vi "实时数据查询用2小时间的数据.vi"(11 "字符串":string) -> (3 "连接的字符串":string)   [LabVIEW 2016, in "数据传输系统-04.lvlib"]
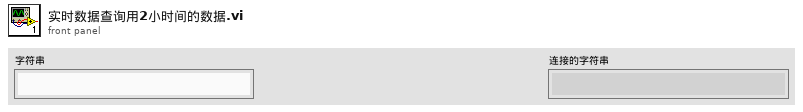
[diagram p1: front panel]
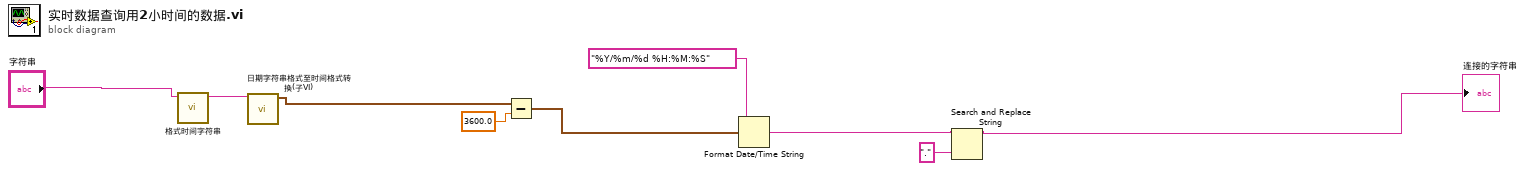
[diagram p0: block diagram]
diagram:
  n1 = call "格式时间字符串.vi"("字符串"="字符串") -> ("连接的字符串"=w2:string)  [unwired: 10 in]
  n2 = call "日期字符串格式至时间格式转换(子VI).vi"("data[0]"=w2) -> ("time stamp"=w1:timestamp)  [unwired: 10 in]
  n3 = Subtract(x=w1, y=3600.0) -> (x-y=w6:timestamp)
  n4 = Format Date/Time String(time format string (%c)="%Y/%m/%d %H:%M:%S" ("格式字符串"), seconds (now)=w6) -> (date/time string=w3:string)  [unwired: 1 in]
  n5 = Search and Replace String(input string=w3, search string="." ("搜索字符串")) -> (result string=→"连接的字符串":string)  [unwired: 6 in, 3 out]
